vi "UpdateControls.vi"(6 "50mA Spectra":cluster{"Wavelength":dbl[], "EL Spectrum":dbl[]}, 8 "error in (no error)":errorcluster, 9 "20mA Spectra":cluster{"Wavelength":dbl[], "EL Spectrum":dbl[]}, 10 "Data In":T1 {"50mA Data"."Reverse" format="%#_3g"; "50mA Data"."Current,mA" format="%_6g"; "50mA Data"."Knee Current" format="%#_3g"; "50mA Data"."WL" format="%_6g"; "50mA Data"."Voltage" format="%_6g"; "50mA Data"."Power" format="%_5g"; "20mA Data"."Reverse" format="%#_3g"; "20mA Data"."Current,mA" format="%_6g"; "20mA Data"."Knee Current" format="%#_3g"; "20mA Data"."WL" format="%_6g"; "20mA Data"."Voltage" format="%_6g"; "20mA Data"."Power" format="%_5g"}, 11 "EpiWrapper in":refnum<class "EpiWrapper.lvclass">) -> (0 "error out":errorcluster, 2 "KneeFail?":bool, 3 "EpiWrapper out":refnum<class "EpiWrapper.lvclass">)   [LabVIEW 2012, in "EpiWrapper.lvclass"]
uses:
  EpiWrapper.lvclass
  Controls/TestData.ctl
  Controls/Measurement.ctl
  EpiWrapper.lvclass/EpiWrapper.ctl
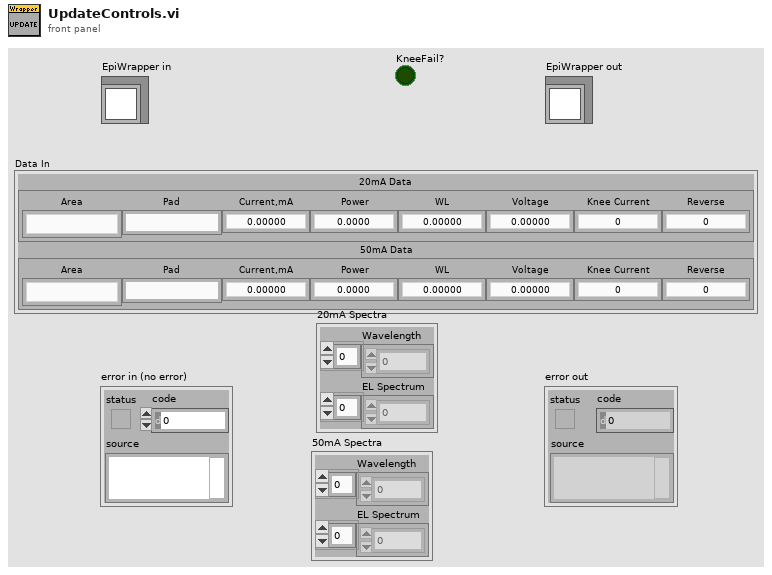
[diagram p1: front panel]
types:
  T1 = typedef "TestData.ctl" = cluster{"20mA Data":T2, "50mA Data ":T2}
  T2 = typedef "Measurement.ctl" = cluster{"Area":string, "Pad":string, "Current,mA":dbl, "Power":dbl, "WL":dbl, "Voltage":dbl, "Knee Current":dbl, "Reverse":dbl}
  T3 = typedef "MeasureControl.ctl" = cluster{"Graph":cluster{"Y":dbl[], "Y":dbl[]}[], "Pass":bool, "Fail":bool, "Measure":bool, "Wafer Area":T4, "TestData":T1, "Pad":string}
  T4 = typedef "PadArea.ctl" = enum16{"A", "B", "C", "D", "L", "R", "T", "G"}
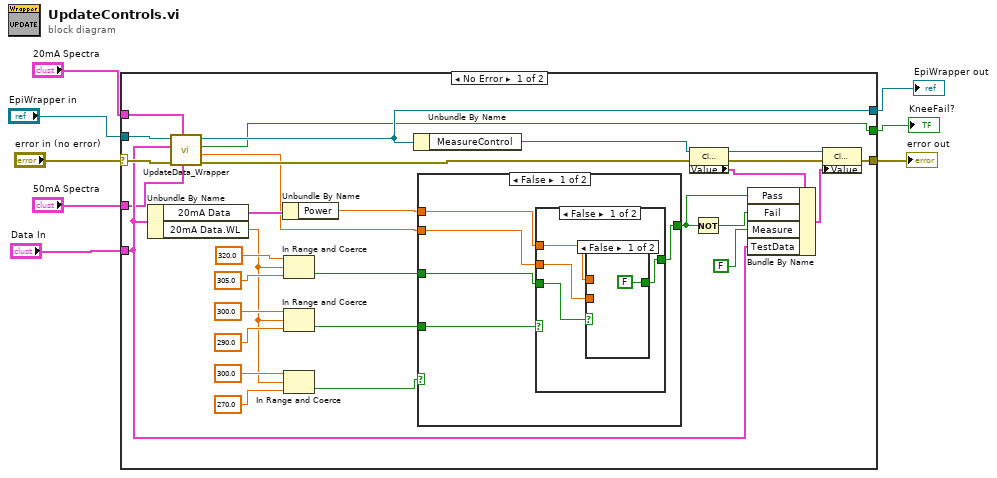
[diagram p0: block diagram]
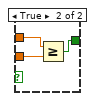
[diagram p2: hidden frame]
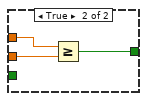
[diagram p3: hidden frame]
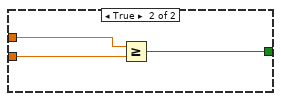
[diagram p4: hidden frame]
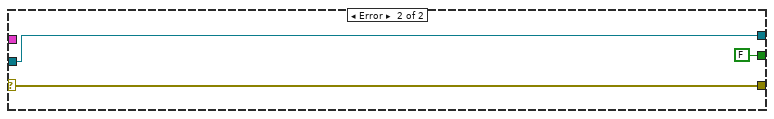
[diagram p5: hidden frame]
diagram:
  n1 = case shown="No Error" "error in (no error)" {
    selector: "error in (no error)" -> [w17 w60]
    tunnel: [w18 w60] -> w7
    tunnel: [w11 w59] -> w6
    tunnel: "EpiWrapper in" -> [w12 w59]
    tunnel: "Data In" -> [w15 _]
    tunnel: "20mA Spectra" -> [w14 _]
    tunnel: "50mA Spectra" -> [w13 _]
    tunnel: [w10 FALSE ("KneeFail?")] -> w1
    frame No Error {
      n2 = Unbundle By Name(w15) -> ("20mA Data"=w36:T2, "20mA Data.WL"=w22:dbl)
      n3 = call-dynamic "UpdateData_Wrapper.vi"("50mA Spectra"=w13, "20mA Spectra"=w14, "error in (no error)"=w17, "Data In"=w15, "EpiWrapper in"=w12) -> ("error out"=w16:errorcluster, "PowerMin"=w9:dbl, "KneeFail?"=w10:bool, "EpiWrapper out"=w11:refnum<class "EpiWrapper.lvclass">)  [unwired: 3 in]
      n4 = Unbundle By Name(w36) -> ("Power"=w26:dbl)
      n5 = In Range and Coerce(upper limit=320.0, x=w22, lower limit=305.0) -> (In Range?=w27:bool)  [unwired: 1 out]
      n6 = In Range and Coerce(upper limit=300.0, x=w22, lower limit=290.0) -> (In Range?=w28:bool)  [unwired: 1 out]
      n7 = In Range and Coerce(upper limit=300.0, x=w22, lower limit=270.0) -> (In Range?=w29:bool)  [unwired: 1 out]
      n8 = Unbundle By Name(w11) -> ("MeasureControl"=w38:refnum<vi>)
      n9 = case shown="False" w29 {
        tunnel: w28 -> [w43 _]
        tunnel: w27 -> [w42 _]
        tunnel: w26 -> [w41 w57]
        tunnel: [w40 w56] -> w23
        tunnel: w9 -> [w39 w55]
        frame False {
          n10 = case shown="False" w43 {
            tunnel: w42 -> [w47 _]
            tunnel: w41 -> [w46 w54]
            tunnel: [w45 w53] -> w40
            tunnel: w39 -> [w44 w52]
            frame False {
              n11 = case shown="False" w47 {
                tunnel: w46 -> [_ w51]
                tunnel: [FALSE w50] -> w45
                tunnel: w44 -> [_ w49]
                frame False {
                }
                frame True {
                  n12 = Greater Or Equal?(x=w51, y=w49) -> (x >= y?=w50:bool)
                }
              }
            }
            frame True {
              n13 = Greater Or Equal?(x=w54, y=w52) -> (x >= y?=w53:bool)
            }
          }
        }
        frame True {
          n14 = Greater Or Equal?(x=w57, y=w55) -> (x >= y?=w56:bool)
        }
      }
      n15 = property class="Clust (strict)"(reference=w38, error in=w16) -> (reference out=w20:refnum<vi>, error out=w19:errorcluster, "Value"=w37:T3)
      n16 = Not(x=w23) -> (.not. x?=w25:bool)
      n17 = Bundle By Name(cluster=w37, "Pass"=w23, "Fail"=w25, "Measure"=FALSE, "TestData"=w15) -> (w21:T3)
      n18 = property class="Clust (strict)"(reference=w20, error in=w19, "Value"=w21) -> (error out=w18:errorcluster)  [unwired: 1 out]
    }
    frame Error {
    }
  }
  "error out" <- w7
  "EpiWrapper out" <- w6
  "KneeFail?" <- w1
